vi "Get Comment.vi"(8 "error in (no error)":errorcluster, 11 "DOM document in":refnum<k20>) -> (0 "error out":errorcluster, 2 "comment":string, 3 "DOM document out":refnum<k20>)   [LabVIEW 2017, in "Error File Management.lvlib"]
uses:
  Error File Management.lvlib
  <vilib>/xml/Close Reference(Node).vi
  <vilib>/xml/NI_XML.lvlib
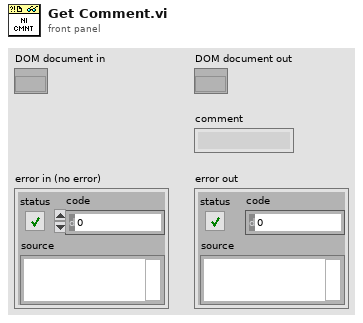
[diagram p1: front panel]
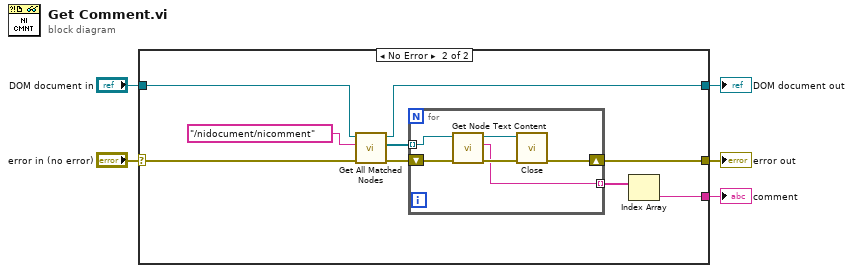
[diagram p0: block diagram]
diagram:
  n1 = case shown="No Error" "error in (no error)" {
    selector: "error in (no error)" -> [w7 w8]
    tunnel: [_ w16] -> w5
    tunnel: [w6 w15] -> w4
    tunnel: "DOM document in" -> [w6 w14]
    tunnel: [w7 w9] -> w1
    frame Error {
    }
    frame No Error {
      n2 = call <vilib>:"Get All Matched Nodes.vi"("error in (no error)"=w8, "XPath expression"="/nidocument/nicomment", "node in"=w14) -> ("error out"=w12:errorcluster, "node result array"=w11:refnum<k20>[], "node out"=w15:refnum<k20>)  [unwired: 6 in]
      n3 = for {
        tunnel: w11 -> [w19] mode=indexing
        tunnel: [w20] -> w13 mode=indexing
        shift-right: [w21] -> w9
        shift-left: w12 -> [w18]
        n4 = call "Get Node Text Content.vi"("error in (no error)"=w18, "node in"=w19) -> ("error out"=w22:errorcluster, "node text"=w20:string, "node out"=w17:refnum<k20>)  [unwired: 7 in]
        n5 = call-poly <vilib>:"Close.vi"("error in (no error)"=w22, "node"=w17) -> ("error out"=w21:errorcluster)  [unwired: 7 out]
      }
      n6 = Index Array(array=w13) -> (element=w16:string)  [unwired: 1 in]
    }
  }
  "comment" <- w5
  "DOM document out" <- w4
  "error out" <- w1
